vi "User Process Test.vi"() -> ()   [LabVIEW 2015, in "Custom Temperature Controller tests.lvlib"]
uses:
  Custom Temperature Controller tests.lvlib
  module/execution/parameter user data.ctl
  module/execution/result user data.ctl
  module/execution/Custom Temperature Controller runtime.lvclass
panel:
  in  "stop":bool
  out "error out":errorcluster
  out "Results from processing":T1
  in  "Parameters to process":T2
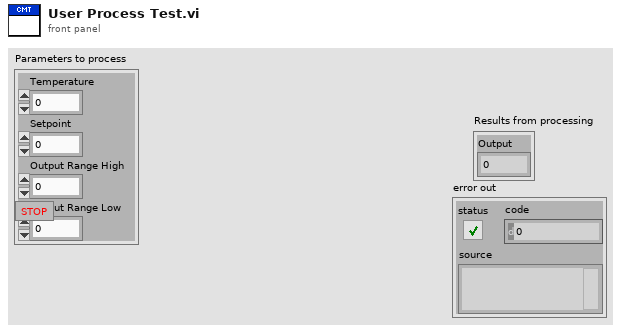
[diagram p1: front panel]
types:
  T1 = typedef "Custom Temperature Controller runtime.lvclass/result user data.ctl" = cluster{"Output":dbl}
  T2 = typedef "Custom Temperature Controller runtime.lvclass/parameter user data.ctl" = cluster{"Temperature":dbl, "Setpoint":dbl, "Output Range High":dbl, "Output Range Low":dbl}
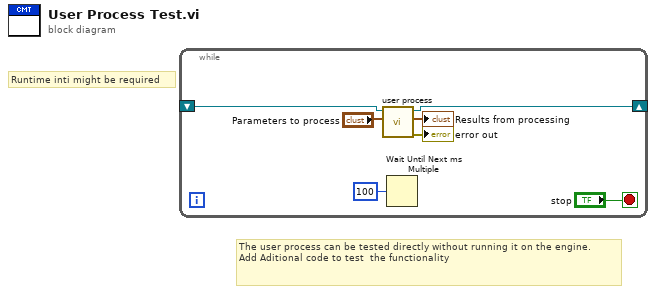
[diagram p0: block diagram]
diagram:
  # "Runtime inti might be required"
  # "The user process can be tested directly without running it on the engine.\nAdd Aditional code to test  the functionality"
  n1 = while {
    shift-right: [w1] -> _
    shift-left: _ -> [w2]
    stop <- "stop" stop-if-true
    n2 = call "user process.vi"("Parameters to process"="Parameters to process", "Custom Temperature Controller runtime in"=w2) -> ("error out"=→"error out":errorcluster, "Results from processing"=→"Results from processing":T1, "Custom Temperature Controller runtime out"=w1:refnum<class "Custom Temperature Controller runtime.lvclass">)  [unwired: 7 in]
    n3 = Wait Until Next ms Multiple(millisecond multiple=u32 100) -> ()  [unwired: 1 out]
  }
